vi "Set Meas Step Values.vi"(8 "error in (no error)":errorcluster, 11 "Skyworks - PVT in":refnum<class "Skyworks - PVT.lvclass">) -> (0 "error out":errorcluster, 3 "Skyworks - PVT out":refnum<class "Skyworks - PVT.lvclass">)   [LabVIEW 2018, in "Skyworks PVT.lvlib" / "Skyworks - PVT.lvclass"]
uses:
  Skyworks - PVT.lvclass
  Plugins/Measurement Interface.lvlibp/Measurement Interface.lvclass
  C:/Sequence Automation/Plugins/Measurement Interface.lvlibp/Measurement Interface.lvclass
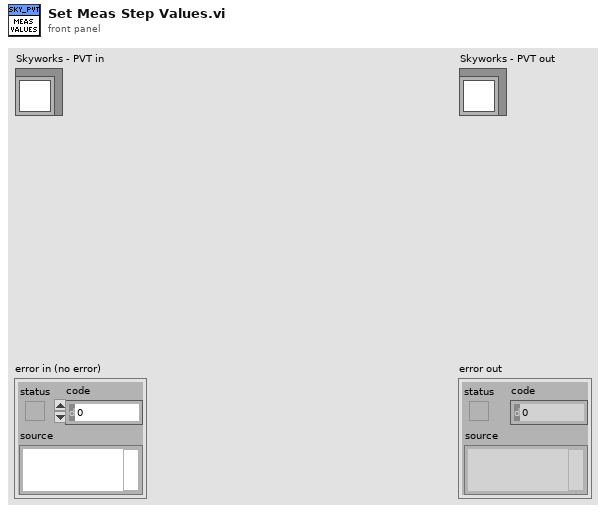
[diagram p1: front panel]
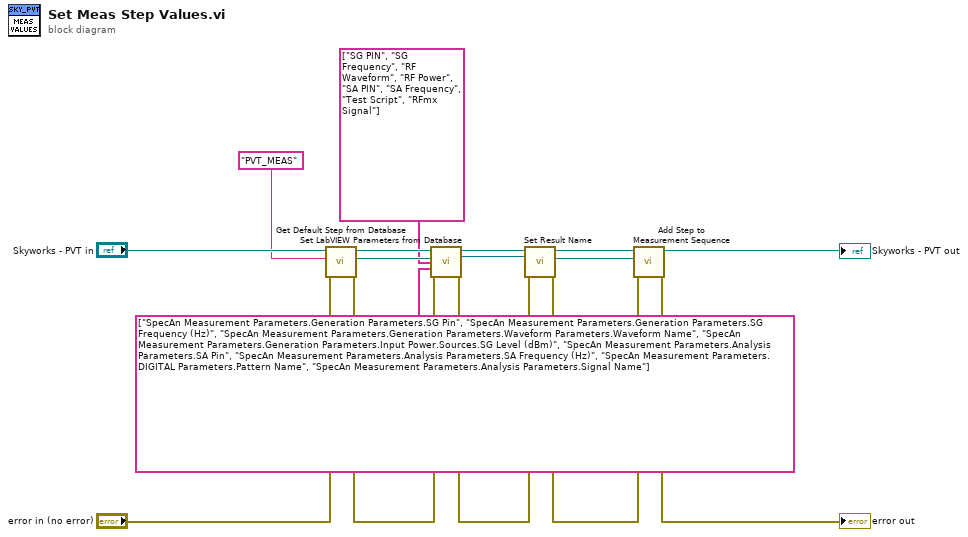
[diagram p0: block diagram]
diagram:
  n1 = call "Get Default Step from Database.vi"("error in (no error)"="error in (no error)", "Default Step"="PVT_MEAS", "Measurement Interface in"="Skyworks - PVT in") -> ("error out"=w14:errorcluster, "Cloned Step"=w7:refnum<k7>, "Measurement Interface out"=w15:refnum<class "Skyworks - PVT.lvclass">)  [unwired: 6 in]
  n2 = call "Set LabVIEW Parameters from Database.vi"("Measurement Interface in"=w15, "Step In"=w7, "Dictionary Keys"=string[] ["SG PIN", "SG Frequency", "RF Waveform", "RF Power", "SA PIN", "SA Frequency", "Test Script", "RFmx Signal"], "LabVIEW Parameter Mapping"=string[] ["SpecAn Measurement Parameters.Generation Parameters.SG Pin", "SpecAn Measurement Parameters.Generation Parameters.SG Frequency (Hz)", "SpecAn Measurement Parameters.Generation Parameters.Waveform Parameters.Waveform Name", "SpecAn Measurement Parameters.Generation Parameters.Input Power.Sources.SG Level (dBm)", "SpecAn Measurement Parameters.Analysis Parameters.SA Pin", "SpecAn Measurement Parameters.Analysis Parameters.SA Frequency (Hz)", "SpecAn Measurement Parameters.DIGITAL Parameters.Pattern Name", "SpecAn Measurement Parameters.Analysis Parameters.Signal Name"], "error in (no error)"=w14) -> ("Measurement Interface out"=w13:refnum<class "Skyworks - PVT.lvclass">, "Step Out"=w3:refnum<k7>, "error out"=w12:errorcluster)  [unwired: 8 in]
  n3 = call "Set Result Name.vi"("error in (no error)"=w12, "Step In"=w3, "Skyworks - PVT in"=w13) -> ("error out"=w10:errorcluster, "Step Out"=w8:refnum<k7>, "Skyworks - PVT out"=w11:refnum<class "Skyworks - PVT.lvclass">)  [unwired: 6 in]
  n4 = call "Add Step to Measurement Sequence.vi"("error in (no error)"=w10, "Step to Add"=w8, "Measurement Interface in"=w11) -> ("error out"=→"error out":errorcluster, "Measurement Interface out"=→"Skyworks - PVT out":refnum<class "Skyworks - PVT.lvclass">)  [unwired: 7 in]
